vi "Set LabVIEW VI Topmost.vi"(8 "error in (no error)":errorcluster, 11 "VI Refnum (null)":refnum<vi>) -> (0 "error out":errorcluster, 2 "Result":string, 3 "dup VI Refnum":refnum<vi>)   [LabVIEW 2011]
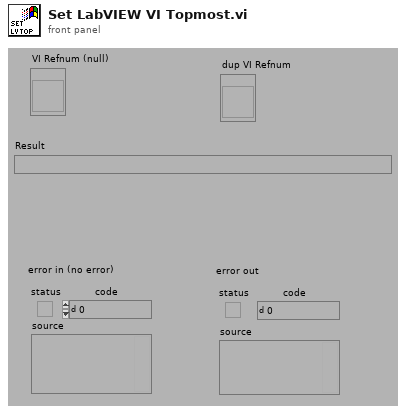
[diagram p1: front panel]
types:
  T1 = enum16{"HWND_TOP", "HWND_BOTTOM", "HWND_TOPMOST", "HWND_NOTOPMOST"}
  T2 = cluster{"SWP_NOSIZE (x1)":bool, "SWP_NOMOVE (x2)":bool, "SWP_NOZORDER (x4)":bool, "SWP_NOREDRAW (x8)":bool, "SWP_NOACTIVATE (x10)":bool, "SWP_DRAWFRAME (x20)":bool, "SWP_SHOWWINDOW (x40)":bool, "SWP_HIDEWINDOW (x80)":bool, "SWP_NOCOPYBITS (x100)":bool, "SWP_NOOWNERZORDER (x200)":bool, "SWP_NOSENDCHANGING (x400)":bool, "SWP_DEFERERASE (x2000)":bool, "SWP_ASYNCWINDOWPOS (x4000)":bool}
  T3 = typedef "hWnd.ctl" = refnum<k1>
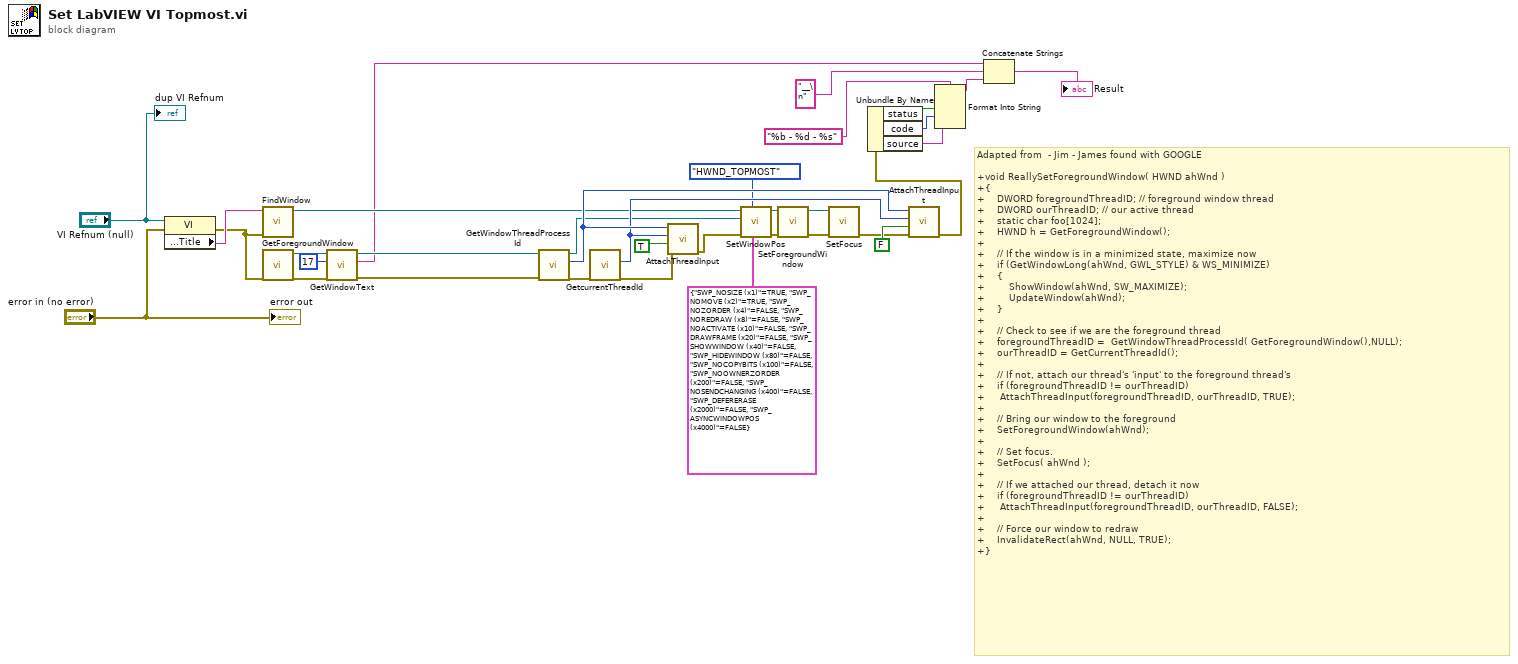
[diagram p0: block diagram]
diagram:
  # "Adapted from  - Jim - James found with GOOGLE\n\n+void ReallySetForegroundWindow( HWND ahWnd )\n+{\n+    DWORD foregroundThreadID; // foreground window thread\n+    DWORD ourThreadID; // our active thread\n+    static char foo[1024];\n+    HWND h = GetForegroundWindow();\n+\n+    // If the window is in a minimized state, maximize now\n+    if (GetWindowLong(ahWnd, GWL_STYLE) & WS_MINIMIZE)\n+    {\n+        ShowWindow(ahWnd, SW_MAXIMIZE);\n+        UpdateWindow(ahWnd);\n+    }\n+\n+    // Check to see if we are the foreground thread\n+    foregroundThreadID =  GetWindowThreadProcessId( GetForegroundWindow(),NULL);\n+    ourThreadID = GetCurrentThreadId();\n+\n+    // If not, attach our thread's 'input' to the foreground thread's\n+    if (foregroundThreadID != ourThreadID)\n+     AttachThreadInput(foregroundThreadID, ourThreadID, TRUE);\n+\n+    // Bring our window to the foreground\n+    SetForegroundWindow(ahWnd);\n+\n+    // Set focus.\n+    SetFocus( ahWnd );\n+\n+    // If we attached our thread, detach it now\n+    if (foregroundThreadID != ourThreadID)\n+     AttachThreadInput(foregroundThreadID, ourThreadID, FALSE);\n+\n+    // Force our window to redraw\n+    InvalidateRect(ahWnd, NULL, TRUE);\n+}"
  n1 = property class="VI"(reference="VI Refnum (null)", error in="error in (no error)") -> (error out=w25:errorcluster, "Front Panel Window:Title"=w26:string)  [unwired: 1 out]
  n2 = call "FindWindow.vi"("error in (no error)"=w25, "window name (\"\")"=w26) -> ("hWnd"=w19:T3)  [unwired: 7 out]
  n3 = call "GetForegroundWindow.vi"("error in (no error)"=w25) -> ("error out"=w15:errorcluster, "dup hWnd"=w14:T3)  [unwired: 9 out]
  n4 = call "GetWindowText.vi"("error in (no error)"=w15, "nMaxCount"=17, "hWnd (NULL)"=w14) -> ("error out"=w11:errorcluster, "window text"=w10:string, "dup hWnd"=w12:T3)  [unwired: 6 out]
  n5 = call "GetWindowThreadProcessId.vi"("error in (no error)"=w11, "hWnd (NULL)"=w12) -> ("error out"=w32:errorcluster, "threadID"=w29:u32, "dup hWnd"=w18:T3)  [unwired: 7 out]
  n6 = call "GetcurrentThreadId.vi"("error in (no error)"=w32) -> ("error out"=w31:errorcluster, "threadID"=w28:u32)  [unwired: 9 out]
  n7 = call "AttachThreadInput.vi"("error in (no error)"=w31, "Fattach"=TRUE, "threadID attach"=w28, "threadID Attachto"=w29) -> ("error out"=w20:errorcluster)  [unwired: 7 out]
  n8 = call "SetWindowPos.vi"("Flags"=T2 {"SWP_NOSIZE (x1)"=TRUE, "SWP_NOMOVE (x2)"=TRUE, "SWP_NOZORDER (x4)"=FALSE, "SWP_NOREDRAW (x8)"=FALSE, "SWP_NOACTIVATE (x10)"=FALSE, "SWP_DRAWFRAME (x20)"=FALSE, "SWP_SHOWWINDOW (x40)"=FALSE, "SWP_HIDEWINDOW (x80)"=FALSE, "SWP_NOCOPYBITS (x100)"=FALSE, "SWP_NOOWNERZORDER (x200)"=FALSE, "SWP_NOSENDCHANGING (x400)"=FALSE, "SWP_DEFERERASE (x2000)"=FALSE, "SWP_ASYNCWINDOWPOS (x4000)"=FALSE}, "hWndInsertAfterALT\n(HWND_TOP)"=T1."HWND_TOPMOST" ("hWndInsertAfterALT\n(HWND_TOP)"), "error in (no error)"=w20, "hWndInsertAfter\n(NULL - use ALT)"=w18, "hWnd (NULL)"=w19) -> ("error out"=w24:errorcluster, "dup hWnd"=w23:T3)  [unwired: 1 in, 4 out]
  n9 = call "SetForegroundWindow.vi"("error in (no error)"=w24, "hWnd (NULL)"=w23) -> ("error out"=w17:errorcluster, "dup hWnd"=w21:T3)  [unwired: 8 out]
  n10 = call "SetFocus.vi"("error in (no error)"=w17, "hWnd (NULL)"=w21) -> ("error out"=w16:errorcluster)  [unwired: 9 out]
  n11 = call "AttachThreadInput.vi"("error in (no error)"=w16, "Fattach"=FALSE, "threadID attach"=w28, "threadID Attachto"=w29) -> ("error out"=w8:errorcluster)  [unwired: 7 out]
  n12 = Unbundle By Name(w8) -> ("status"=w7:bool, "code"=w6:i32, "source"=w5:string)
  n13 = Format Into String(format string="%b - %d - %s" ("string"), w7, w6, w5) -> (resulting string=w4:string)  [unwired: 2 in, 1 out]
  n14 = Concatenate Strings(w10, "__\n" ("string"), w4) -> (→"Result":string)
  "error out" <- "error in (no error)"
  "dup VI Refnum" <- "VI Refnum (null)"
